vi "VsEP-Create Stimuli.vi"(0 "Runtime":T1, 7 "Hidden":T2, 11 "error in (no error)":errorcluster) -> (8 "VsEP stimuli":dbl[][](array[numeric]), 15 "error out":errorcluster)   [LabVIEW 2020]
uses:
  Typedefs/VsEP-Hidden Params.ctl
  epl-vi-lib/Signal Synthesis VIs/Controls/Gate XCtl/Gate Control.xctl
  Typedefs/VsEP-Runtime Data.ctl
  epl-vi-lib/Utility VIs/Math VIs/dB to Linear (scalar).vi
  epl-vi-lib/PXI DAQ VIs/DAQ Engine VIs/PXI Globals.vi
panel:
  out "Waveform Graph":dbl[][](graph)
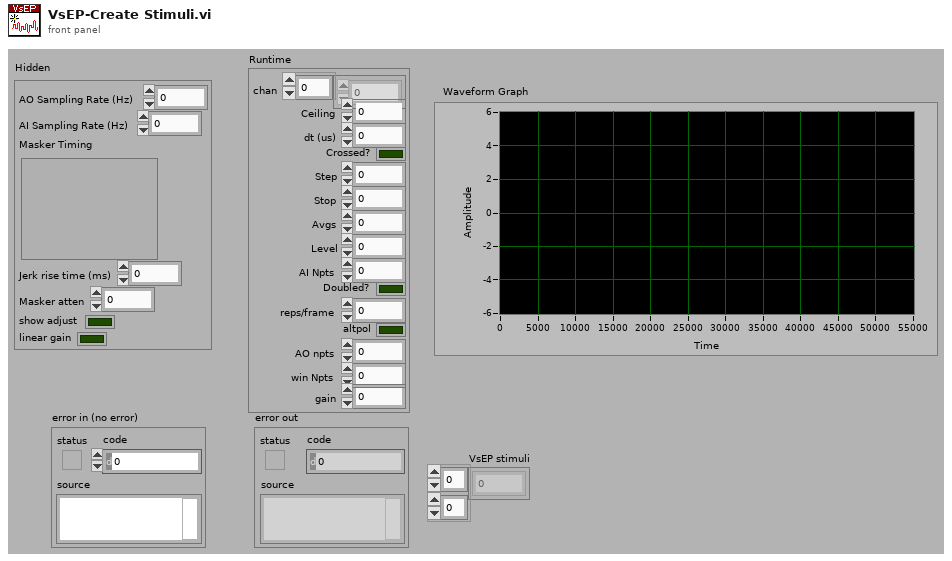
[diagram p1: front panel]
types:
  T1 = typedef "VsEP-Runtime Data.ctl" = cluster{"chan":i32[], "Ceiling":dbl, "dt (us)":dbl, "Crossed?":bool, "Step":dbl, "Stop":i32, "Avgs":i32, "Level":dbl, "AI Npts":i32, "Doubled?":bool, "reps/frame":i32, "altpol":bool, "AO npts":i32, "win Npts":i32, "gain":dbl}
  T2 = typedef "VsEP-Hidden Params.ctl" = cluster{"AO Sampling Rate (Hz)":dbl, "AI Sampling Rate (Hz)":dbl, "Masker Timing":cluster{"Active":bool, "Delay (ms)":dbl, "Width (ms)":dbl, "Ramp (ms)":dbl}, "Jerk rise time (ms)":dbl, "Masker atten":dbl, "show adjust":bool, "linear gain":bool}
  T3 = cluster{"Active":bool, "Delay (ms)":dbl, "Width (ms)":dbl, "Ramp (ms)":dbl}
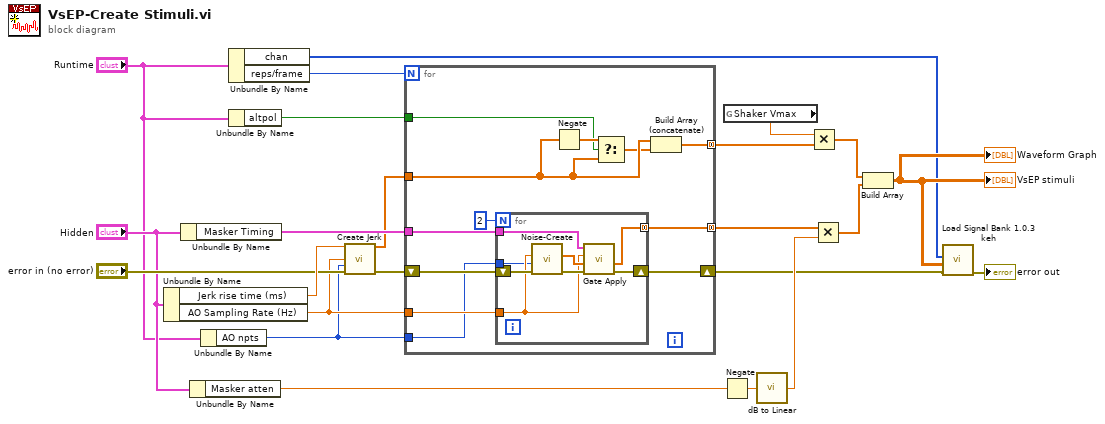
[diagram p0: block diagram]
diagram:
  n1 = Unbundle By Name("Hidden") -> ("Jerk rise time (ms)"=w23:dbl, "AO Sampling Rate (Hz)"=w16:dbl)
  n2 = Unbundle By Name("Hidden") -> ("Masker Timing"=w20:T3)
  n3 = Unbundle By Name("Hidden") -> ("Masker atten"=w10:dbl)
  n4 = Unbundle By Name("Runtime") -> ("AO npts"=w1:i32)
  n5 = Unbundle By Name("Runtime") -> ("chan"=w2:i32[], "reps/frame"=w11:i32)
  n6 = Unbundle By Name("Runtime") -> ("altpol"=w12:bool)
  n7 = call "Create Jerk.vi"("Rise time (ms)"=w23, "Sampling Rate (Hz)"=w16, "Npts"=w1, "error in (no error)"="error in (no error)") -> ("Waveform"=w19:dbl[], "error out"=w21:errorcluster)  [unwired: 10 in]
  n8 = for {
    N: w11 -> [_]
    tunnel: w20 -> [w34]
    tunnel: w19 -> [w31]
    tunnel: [w29] -> w18 mode=concatenating
    tunnel: [w28] -> w17 mode=concatenating
    tunnel: w16 -> [w27]
    tunnel: w12 -> [w26]
    shift-right: [w33] -> w5
    shift-left: w21 -> [w35]
    tunnel: w1 -> [w25]
    n9 = for {
      N: 2 -> [_]
      tunnel: w34 -> [w40]
      tunnel: [w38] -> w29 mode=concatenating
      tunnel: w27 -> [w37]
      tunnel: w25 -> [w36]
      shift-right: [w39] -> w33
      shift-left: w35 -> [w43]
      n10 = call "Noise-Create.vi"("error in (no error)"=w43, "Npts"=w36, "Sampling Rate (Hz)"=w37) -> ("error out"=w41:errorcluster, "Waveform"=w42:dbl[])  [unwired: 6 in, 1 out]
      n11 = call "Gate Apply.vi"("error in (no error)"=w41, "Waveform in"=w42, "Sampling Rate (Hz)"=w37, "Gate Control"=w40) -> ("error out"=w39:errorcluster, "Gated waveform"=w38:dbl[])  [unwired: 6 in]
    }
    n12 = Negate(x=w31) -> (-x=w32:dbl[])
    n13 = Select(t=w32, s=w26, f=w31) -> (s? t:f=w30:dbl[])
    n14 = Build Array (concatenate)(w31, w30) -> (w28:dbl[])
  }
  n15 = Negate(x=w10) -> (-x=w14:dbl)
  n16 = global read "PXI Globals.vi" "Shaker Vmax"() -> (w6:dbl)
  n17 = call-poly "dB to Linear.vi"("dB"=w14) -> ("linear"=w13:dbl)
  n18 = Multiply(x=w6, y=w17) -> (x*y=w7:dbl[])
  n19 = Multiply(x=w18, y=w13) -> (x*y=w15:dbl[])
  n20 = Build Array(w7, w15) -> (w4:dbl[][])
  "VsEP stimuli" <- w4
  "Waveform Graph" <- w4
  n21 = call "Load Signal Bank 1.0.3 keh.vi"("error in (no error)"=w5, "Input array"=w4, "Active AO Array"=w2) -> ("error out"=→"error out":errorcluster)  [unwired: 6 in, 2 out]
